vi "Stop Core.vi"(10 "final error code":i32, 11 "Measure Object in":refnum<class "Worker Actor.lvclass">) -> (3 "Measure Object out":refnum<class "Worker Actor.lvclass">)   [LabVIEW 2024, in "Worker Actor.lvclass"]
doc: "(<B>Filename</B>: Actor Framework.lvlib:Actor.lvclass:Stop Core.vi)\n\nDefines what the actor does before it stops. Use the <B>final error code</B> input to determine whether the actor shut down in response to an error.\n\nBy default, this method does nothing. A descendant class may override it to define behavior, such as shutting down any processes the actor initiated in its override of the Actor Core method."
uses:
  Worker Actor.lvclass
  Worker Actor.lvclass/Worker Actor.ctl
  Template Module/Read State.vi
  Template Module/Template Module.lvclass
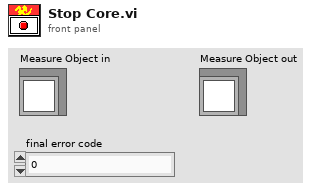
[diagram p1: front panel]
types:
  T1 = typedef "Worker State.ctl" = enum16{"Idle", "Starting", "Working", "Stopping"}
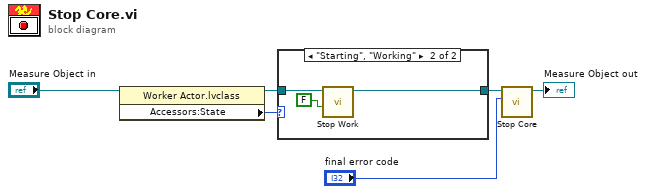
[diagram p0: block diagram]
diagram:
  n1 = property class="Worker Actor.lvclass"(reference="Measure Object in") -> (reference out=w3:refnum<class "Worker Actor.lvclass">, "Accessors:State"=w1:T1)  [unwired: 1 in, 1 out]
  n2 = case shown="\"Starting\", \"Working\"" w1 {
    tunnel: w3 -> [w7 w10]
    tunnel: [w7 w9] -> w2
    frame "Idle", Default {
    }
    frame "Starting", "Working" {
      n3 = call-dynamic "Stop Work.vi"("Reply"=FALSE, "Worker in"=w10) -> ("Worker out"=w9:refnum<class "Worker Actor.lvclass">)  [unwired: 8 in, 1 out]
    }
  }
  n4 = call-parent "Stop Core.vi"("final error code"="final error code", "Measure Object in"=w2) -> ("Measure Object out"=→"Measure Object out":refnum<class "Worker Actor.lvclass">)  [unwired: 9 in]
